vi "Insert Demo Data.vi"() -> ()   [LabVIEW 2014, in "DB-Configuration.lvlib"]
doc: "This VI inserts demo data into oracle database configuration tables"
uses:
  DB-Configuration.lvlib
  <vilib>/addons/database/Auxilliary.llb/DB Tools Transaction.ctl
  <vilib>/addons/database/Connection.llb/DB Tools Open Connec (String).vi
  <vilib>/addons/database/Connection.llb/Conn Transaction.vi
  <vilib>/addons/database/NI_Database_API.lvlib
panel:
  in  "Project Path":path
  out "OK?":bool
  # "Insert demo configuration data in Oracle"
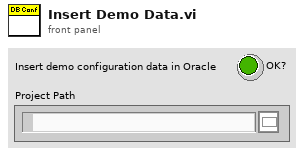
[diagram p1: front panel]
types:
  T1 = typedef "NI_Database_API.lvlib/DB Tools Transaction.ctl" = enum16{"begin", "commit", "rollback"}
  T2 = cluster{"FK_SECTIONS_ID":i32, "FK_ITEMS_ID":i32, "Data":string}[]
  T3 = cluster{"NAME":string, "FK_CLASSES_ID":i32, "FK_BASECLASS":i32}[]
  T4 = cluster{"NAME":string, "PATH":string, "ANCHESTOR":i32}[]
  T5 = typedef "NI_Database_API.lvlib/Conn ObjectReference.ctl" = refnum<k1>
  T6 = cluster{i32, "NAME":string, string, "ANCHESTOR":i32}
  T7 = cluster{i32, "NAME":string, "FK_CLASSES_ID":i32, "FK_BASECLASS":i32}
  T8 = cluster{i32, "FK_SECTIONS_ID":i32, "FK_ITEMS_ID":i32, "Data":string}
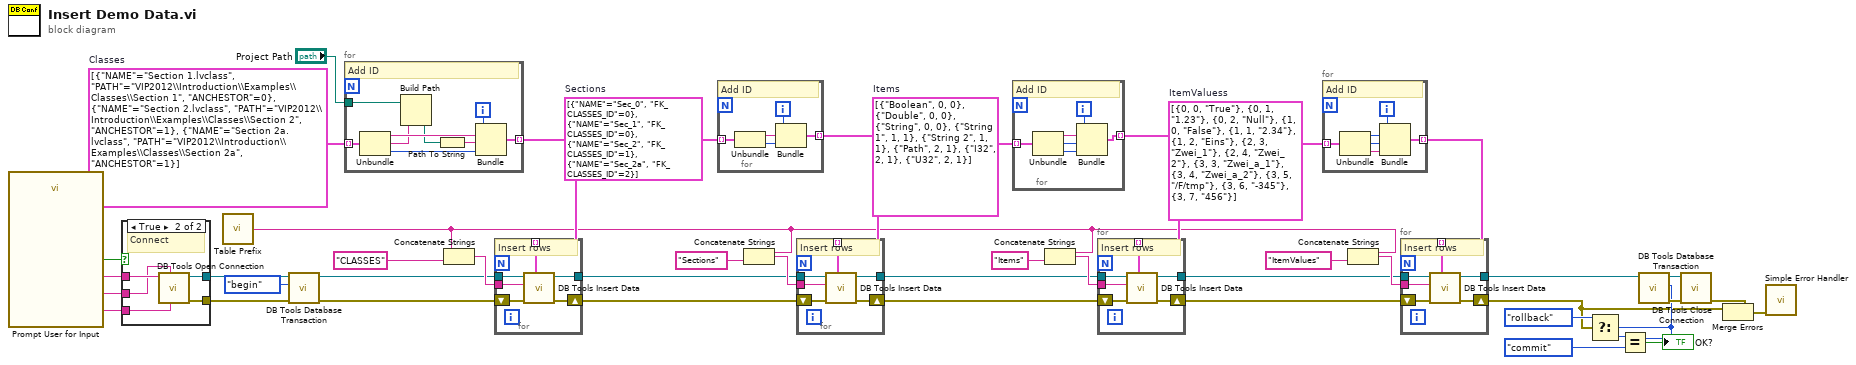
[diagram p0: block diagram]
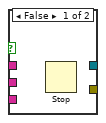
[diagram p2: hidden frame]
diagram:
  w11 = DB_Tools_Transaction."commit" ("operation (begin)")
  w26 = T2 [{"FK_SECTIONS_ID"=0, "FK_ITEMS_ID"=0, "Data"="True"}, {"FK_SECTIONS_ID"=0, "FK_ITEMS_ID"=1, "Data"="1.23"}, {"FK_SECTIONS_ID"=0, "FK_ITEMS_ID"=2, "Data"="Null"}, {"FK_SECTIONS_ID"=1, "FK_ITEMS_ID"=0, "Data"="False"}, {"FK_SECTIONS_ID"=1, "FK_ITEMS_ID"=1, "Data"="2.34"}, {"FK_SECTIONS_ID"=1, "FK_ITEMS_ID"=2, "Data"="Eins"}, {"FK_SECTIONS_ID"=2, "FK_ITEMS_ID"=3, "Data"="Zwei_1"}, {"FK_SECTIONS_ID"=2, "FK_ITEMS_ID"=4, "Data"="Zwei_2"}, {"FK_SECTIONS_ID"=3, "FK_ITEMS_ID"=3, "Data"="Zwei_a_1"}, {"FK_SECTIONS_ID"=3, "FK_ITEMS_ID"=4, "Data"="Zwei_a_2"}, {"FK_SECTIONS_ID"=3, "FK_ITEMS_ID"=5, "Data"="/F/tmp"}, {"FK_SECTIONS_ID"=3, "FK_ITEMS_ID"=6, "Data"="-345"}, {"FK_SECTIONS_ID"=3, "FK_ITEMS_ID"=7, "Data"="456"}]  # ItemValuess
  w33 = T3 [{"NAME"="Boolean", "FK_CLASSES_ID"=0, "FK_BASECLASS"=0}, {"NAME"="Double", "FK_CLASSES_ID"=0, "FK_BASECLASS"=0}, {"NAME"="String", "FK_CLASSES_ID"=0, "FK_BASECLASS"=0}, {"NAME"="String 1", "FK_CLASSES_ID"=1, "FK_BASECLASS"=1}, {"NAME"="String 2", "FK_CLASSES_ID"=1, "FK_BASECLASS"=1}, {"NAME"="Path", "FK_CLASSES_ID"=2, "FK_BASECLASS"=1}, {"NAME"="I32", "FK_CLASSES_ID"=2, "FK_BASECLASS"=1}, {"NAME"="U32", "FK_CLASSES_ID"=2, "FK_BASECLASS"=1}]  # Items
  w36 = cluster{"NAME":string, "FK_CLASSES_ID":i32}[] [{"NAME"="Sec_0", "FK_CLASSES_ID"=0}, {"NAME"="Sec_1", "FK_CLASSES_ID"=0}, {"NAME"="Sec_2", "FK_CLASSES_ID"=1}, {"NAME"="Sec_2a", "FK_CLASSES_ID"=2}]  # Sections
  w42 = T4 [{"NAME"="Section 1.lvclass", "PATH"="VIP2012\\Introduction\\Examples\\Classes\\Section 1", "ANCHESTOR"=0}, {"NAME"="Section 2.lvclass", "PATH"="VIP2012\\Introduction\\Examples\\Classes\\Section 2", "ANCHESTOR"=1}, {"NAME"="Section 2a.lvclass", "PATH"="VIP2012\\Introduction\\Examples\\Classes\\Section 2a", "ANCHESTOR"=1}]  # Classes
  n1 = call "Prompt User for Input"() -> ("Password"=w19:string, "User Name"=w20:string, "ODBC Name"=w21:string, "OK"=w18:bool)  [unwired: 15 in, 1 out]
  n2 = case shown="True" w18 {
    tunnel: w21 -> [_ w48]
    tunnel: w20 -> [_ w47]
    tunnel: w19 -> [_ w46]
    tunnel: [_ w45] -> w5
    tunnel: [_ w44] -> w3
    frame False {
      n3 = Stop() -> ()  [unwired: 1 in]
    }
    frame True {
      # "Connect"
      n4 = call-poly <vilib>:"DB Tools Open Connection.vi"("password"=w46, "userID"=w47, "connection information"=w48) -> ("error out"=w44:errorcluster, "connection reference"=w45:T5)  [unwired: 5 in]
    }
  }
  n5 = call "Table Prefix.vi"() -> ("DB Table Prefix"=w17:string)
  n6 = call-poly <vilib>:"DB Tools Database Transaction.vi"("error in (no error)"=w3, "operation (begin)"=DB_Tools_Transaction."begin", "connection reference"=w5) -> ("error out"=w4:errorcluster, "connection reference out"=w6:T5)  [unwired: 3 in]
  n7 = for {
    tunnel: w42 -> [w57] mode=indexing
    tunnel: [w56] -> w41 mode=indexing
    tunnel: "Project Path" -> [w49]
    i -> [w52]
    # "Add ID"
    n8 = Unbundle(w57) -> ("NAME"=w55:string, "PATH"=w51:string, "ANCHESTOR"=w53:i32)
    n9 = Build Path(base path=w49, name or relative path=w51) -> (appended path=w50:path)
    n10 = Path To String(path=w50) -> (string=w54:string)
    n11 = Bundle(w52, "NAME"=w55, w54, "ANCHESTOR"=w53) -> (w56:T6)  [unwired: 1 in]
  }
  n12 = Concatenate Strings(w17, "CLASSES" ("string")) -> (w22:string)
  n13 = for {
    tunnel: [w63] -> w38
    tunnel: w6 -> [w62]
    tunnel: w22 -> [w59]
    tunnel: w41 -> [w58] mode=indexing
    shift-right: [w61] -> w37
    shift-left: w4 -> [w60]
    # "Insert rows"
    n14 = call <vilib>:"DB Tools Insert Data.vi"("data"=w58, "error in (no error)"=w60, "table"=w59, "connection reference"=w62) -> ("error out"=w61:errorcluster, "connection reference out"=w63:T5)  [unwired: 6 in]
  }
  n15 = for {
    tunnel: w36 -> [w68] mode=indexing
    tunnel: [w66] -> w35 mode=indexing
    i -> [w67]
    # "Add ID"
    n16 = Unbundle(w68) -> ("NAME"=w65:string, "FK_CLASSES_ID"=w64:i32)
    n17 = Bundle(w67, "NAME"=w65, "FK_CLASSES_ID"=w64) -> (w66:cluster{i32, "NAME":string, "FK_CLASSES_ID":i32})  [unwired: 1 in]
  }
  n18 = Concatenate Strings(w17, "Sections" ("string")) -> (w40:string)
  n19 = for {
    tunnel: [w74] -> w30
    tunnel: w38 -> [w73]
    tunnel: w40 -> [w70]
    tunnel: w35 -> [w69] mode=indexing
    shift-right: [w72] -> w29
    shift-left: w37 -> [w71]
    # "Insert rows"
    n20 = call <vilib>:"DB Tools Insert Data.vi"("data"=w69, "error in (no error)"=w71, "table"=w70, "connection reference"=w73) -> ("error out"=w72:errorcluster, "connection reference out"=w74:T5)  [unwired: 6 in]
  }
  n21 = for {
    tunnel: w33 -> [w80] mode=indexing
    tunnel: [w78] -> w34 mode=indexing
    i -> [w79]
    # "Add ID"
    n22 = Unbundle(w80) -> ("NAME"=w77:string, "FK_CLASSES_ID"=w75:i32, "FK_BASECLASS"=w76:i32)
    n23 = Bundle(w79, "NAME"=w77, "FK_CLASSES_ID"=w75, "FK_BASECLASS"=w76) -> (w78:T7)  [unwired: 1 in]
  }
  n24 = Concatenate Strings(w17, "Items" ("string")) -> (w31:string)
  n25 = for {
    tunnel: [w86] -> w24
    tunnel: w30 -> [w85]
    tunnel: w31 -> [w82]
    tunnel: w34 -> [w81] mode=indexing
    shift-right: [w84] -> w23
    shift-left: w29 -> [w83]
    # "Insert rows"
    n26 = call <vilib>:"DB Tools Insert Data.vi"("data"=w81, "error in (no error)"=w83, "table"=w82, "connection reference"=w85) -> ("error out"=w84:errorcluster, "connection reference out"=w86:T5)  [unwired: 6 in]
  }
  n27 = for {
    tunnel: w26 -> [w92] mode=indexing
    tunnel: [w90] -> w25 mode=indexing
    i -> [w91]
    # "Add ID"
    n28 = Unbundle(w92) -> ("FK_SECTIONS_ID"=w89:i32, "FK_ITEMS_ID"=w88:i32, "Data"=w87:string)
    n29 = Bundle(w91, "FK_SECTIONS_ID"=w89, "FK_ITEMS_ID"=w88, "Data"=w87) -> (w90:T8)  [unwired: 1 in]
  }
  n30 = Concatenate Strings(w17, "ItemValues" ("string")) -> (w28:string)
  n31 = for {
    tunnel: [w98] -> w8
    tunnel: w24 -> [w97]
    tunnel: w28 -> [w94]
    tunnel: w25 -> [w93] mode=indexing
    shift-right: [w96] -> w7
    shift-left: w23 -> [w95]
    # "Insert rows"
    n32 = call <vilib>:"DB Tools Insert Data.vi"("data"=w93, "error in (no error)"=w95, "table"=w94, "connection reference"=w97) -> ("error out"=w96:errorcluster, "connection reference out"=w98:T5)  [unwired: 6 in]
  }
  n33 = Select(t=DB_Tools_Transaction."rollback" ("operation (begin)"), s=w7, f=w11) -> (s? t:f=w12:T1)
  n34 = Equal?(x=w12, y=w11) -> (x = y?=→"OK?":bool)
  n35 = call-poly <vilib>:"DB Tools Database Transaction.vi"("operation (begin)"=w12, "connection reference"=w8) -> ("error out"=w15:errorcluster, "connection reference out"=w16:T5)  [unwired: 4 in]
  n36 = call <vilib>:"DB Tools Close Connection.vi"("error in (no error)"=w15, "connection reference"=w16) -> ("error out"=w9:errorcluster)  [unwired: 5 in]
  n37 = Merge Errors(w7, w9) -> (w13:errorcluster)
  n38 = call <vilib>:"Simple Error Handler.vi"("error in (no error)"=w13) -> ()  [unwired: 4 in, 5 out]
